vi "CreateExperimentLogString.vi"(11 "Experiment Log Data Queue Elements":T1[](array[typedef])) -> (3 "Experiment Log String":string)   [LabVIEW 2012]
uses:
  ExperimentLogData.ctl
  ExperimentData.ctl
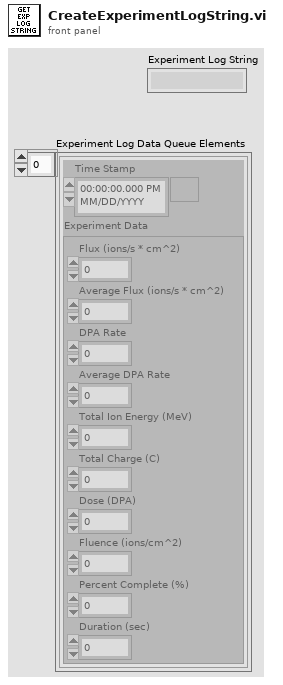
[diagram p1: front panel]
types:
  T1 = typedef "ExperimentLogData.ctl" = cluster{"Time Stamp":timestamp, "Experiment Data":T2}
  T2 = typedef "ExperimentData.ctl" = cluster{"Flux (ions/s * cm^2)":dbl, "Average Flux (ions/s * cm^2)":dbl, "DPA Rate":dbl, "Average DPA Rate":dbl, "Total Ion Energy (MeV)":dbl, "Total Charge (C)":dbl, "Dose (DPA)":dbl, "Fluence (ions/cm^2)":dbl, "Percent Complete (%)":dbl, "Duration (sec)":dbl}
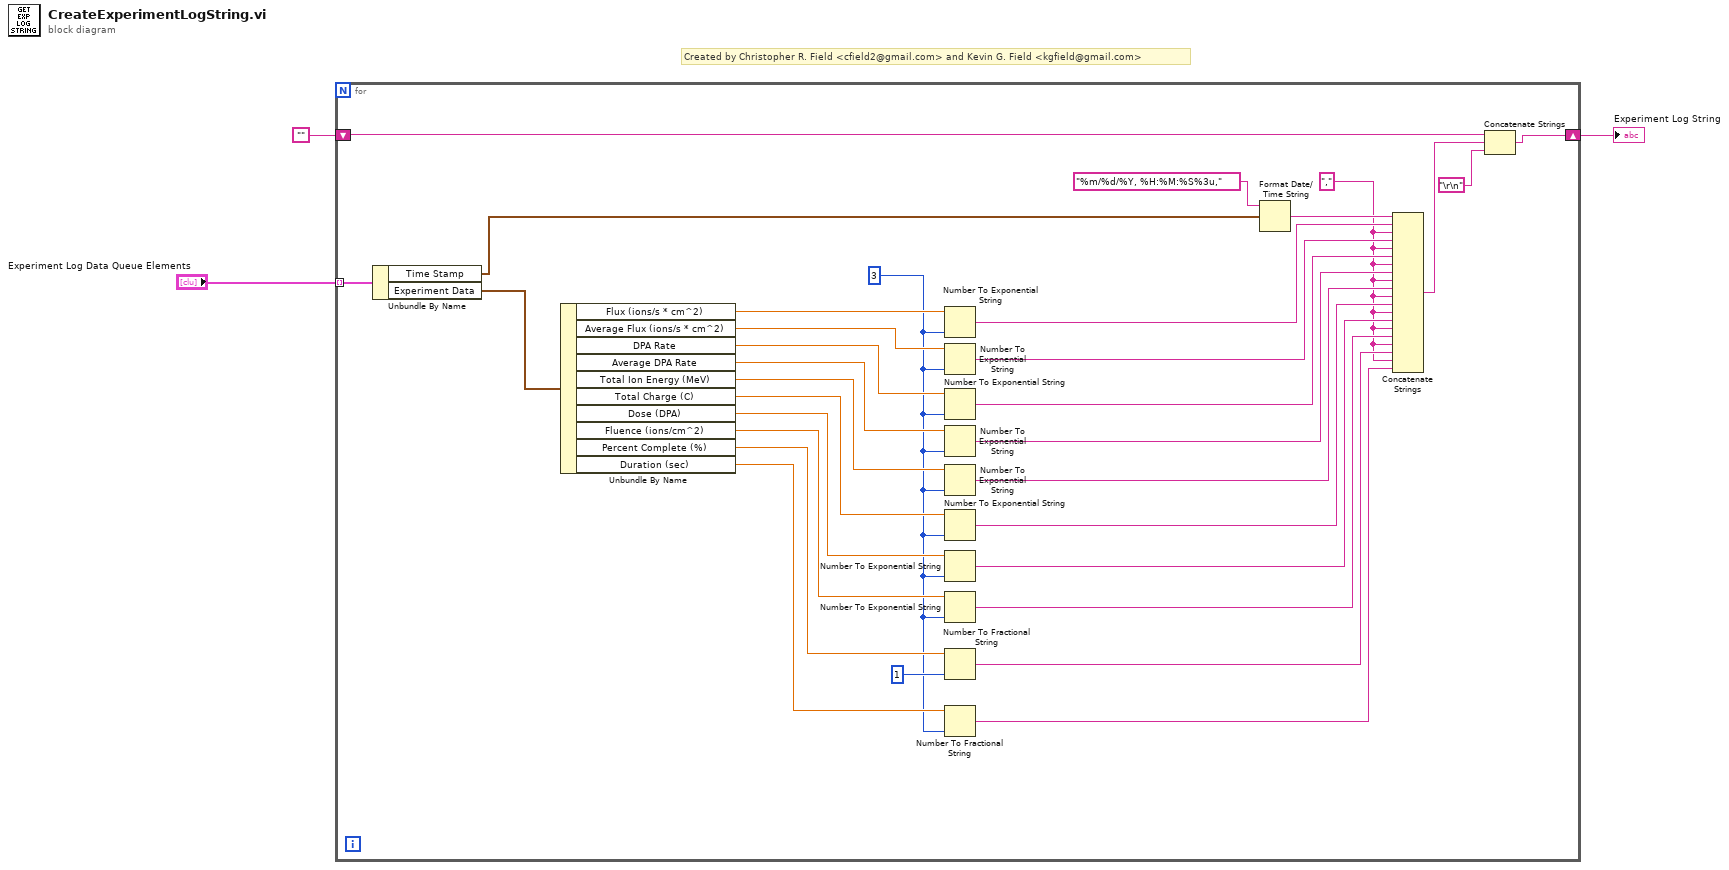
[diagram p0: block diagram]
diagram:
  # "Created by Christopher R. Field <cfield2@gmail.com> and Kevin G. Field <kgfield@gmail.com>"
  n1 = for {
    shift-right: [w30] -> w2
    shift-left: "" -> [w33]
    tunnel: "Experiment Log Data Queue Elements" -> [w29] mode=indexing
    w10 = i16 3 ("precision (6)")
    w5 = ","
    n2 = Unbundle By Name(w29) -> ("Time Stamp"=w27:timestamp, "Experiment Data"=w28:T2)
    n3 = Unbundle By Name(w28) -> ("Flux (ions/s * cm^2)"=w26:dbl, "Average Flux (ions/s * cm^2)"=w24:dbl, "DPA Rate"=w22:dbl, "Average DPA Rate"=w20:dbl, "Total Ion Energy (MeV)"=w18:dbl, "Total Charge (C)"=w16:dbl, "Dose (DPA)"=w15:dbl, "Fluence (ions/cm^2)"=w14:dbl, "Percent Complete (%)"=w13:dbl, "Duration (sec)"=w11:dbl)
    n4 = Number To Exponential String(number=w26, precision (6)=w10) -> (E-format string=w25:string)  [unwired: 2 in]
    n5 = Number To Exponential String(number=w24, precision (6)=w10) -> (E-format string=w23:string)  [unwired: 2 in]
    n6 = Number To Exponential String(number=w22, precision (6)=w10) -> (E-format string=w21:string)  [unwired: 2 in]
    n7 = Number To Exponential String(number=w20, precision (6)=w10) -> (E-format string=w19:string)  [unwired: 2 in]
    n8 = Number To Exponential String(number=w18, precision (6)=w10) -> (E-format string=w17:string)  [unwired: 2 in]
    n9 = Number To Exponential String(number=w16, precision (6)=w10) -> (E-format string=w9:string)  [unwired: 2 in]
    n10 = Number To Exponential String(number=w15, precision (6)=w10) -> (E-format string=w8:string)  [unwired: 2 in]
    n11 = Number To Exponential String(number=w14, precision (6)=w10) -> (E-format string=w7:string)  [unwired: 2 in]
    n12 = Number To Fractional String(number=w13, precision (6)=i16 1) -> (F-format string=w6:string)  [unwired: 2 in]
    n13 = Number To Fractional String(number=w11, precision (6)=w10) -> (F-format string=w4:string)  [unwired: 2 in]
    n14 = Format Date/Time String(time format string (%c)="%m/%d/%Y, %H:%M:%S%3u,", seconds (now)=w27) -> (date/time string=w34:string)  [unwired: 1 in]
    n15 = Concatenate Strings(w34, w25, w5, w23, w5, w21, w5, w19, w5, w17, w5, w9, w5, w8, w5, w7, w5, w6, w5, w4) -> (w32:string)
    n16 = Concatenate Strings(w33, w32, "\r\n") -> (w30:string)
  }
  "Experiment Log String" <- w2
